vi "USB RAW - Bulk.vi"(6 "error in (no error)":errorcluster, 7 "Bulk Out Buffer":string="*IDN?\n", 8 "Bytes To Read":u32=512, 9 "USB RAW VISA resource name":refnum<visa-resource-name>) -> (0 "error out":errorcluster, 2 "Bulk In Buffer":string)   [LabVIEW 2012]
doc: "This example shows how to read and write simple user events from and to a USB RAW device. \n\n<b>Note:</b> This example works only with USB RAW devices.\n\nBefore you run this VI, install a USB RAW device and configure NI Measurement & Automation Explorer (MAX) to recognize the USB device. You can read to and write from the USB RAW device only after you install and configure the USB RAW device and open a session to the device. To read to or write from another device, close the session to the current device, select another device from the <b>USB RAW VISA resource name</b> pull-down menu, and open a session to the new device. \n\nWhen you complete the read or write, click the <b>Stop</b> button to stop the VI."
panel:
  in  "Clear 2":bool
  in  "Stop":bool
  in  "Clear":bool
  in  "BulkIn":bool
  in  "BulkOut":bool
  in  "CloseSession":bool
  in  "OpenSession":bool
  # "On Windows/Linux, consider using the Instrument Driver Finder (Help>>Find Instrument Drivers) to search for an instrument driver for your instrument."
  # "Select Help>>Show Context Help and move the cursor over the VI icon to display help for this VI."
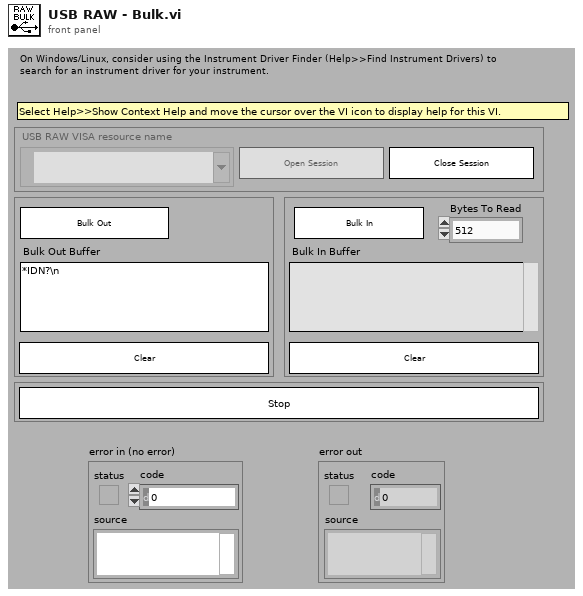
[diagram p1: front panel]
types:
  T1 = enum16{"Initialize/Session Closed", "Session Opened", "Do Nothing"}
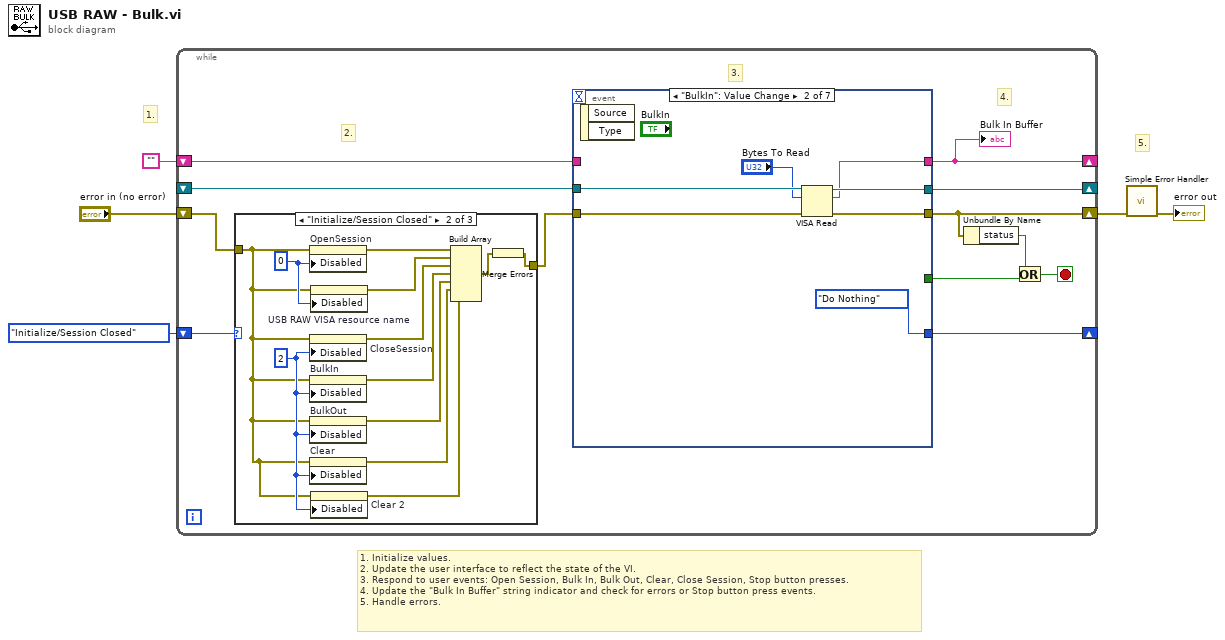
[diagram p0: block diagram]
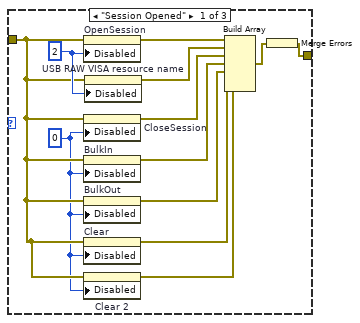
[diagram p2: hidden frame]
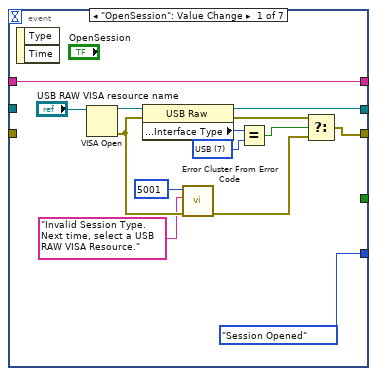
[diagram p4: hidden frame]
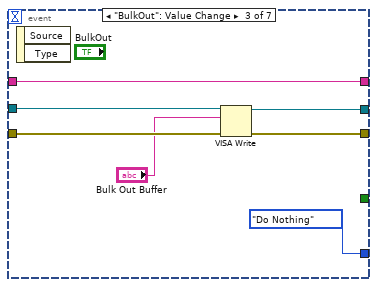
[diagram p5: hidden frame]
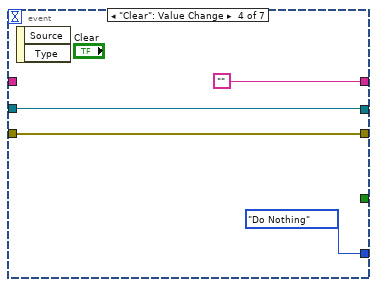
[diagram p6: hidden frame]
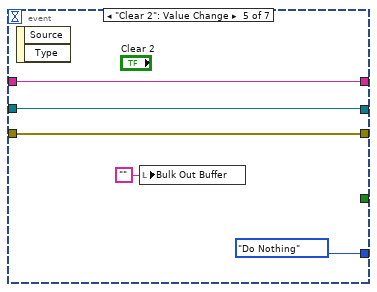
[diagram p7: hidden frame]
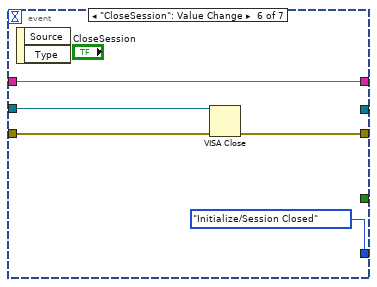
[diagram p8: hidden frame]
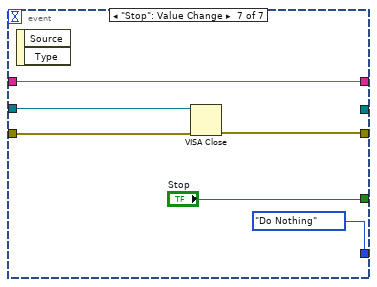
[diagram p9: hidden frame]
diagram:
  # "5."
  # "1."
  # "1. Initialize values.\n2. Update the user interface to reflect the state of the VI.\n3. Respond to user events: Open Session, Bulk In, Bulk Out, Clear, Close Session, Stop button presses.\n4. Update the \"Bulk In Buffer\" string indicator and check for errors or Stop button press events.\n5. Handle errors."
  n1 = while {
    shift-right: [w15] -> _
    shift-left: "" -> [w17]
    shift-right: [w16] -> w3
    shift-left: "error in (no error)" -> [w7]
    shift-right: [w11] -> _
    shift-left: _ -> [w10]
    shift-right: [w6] -> _
    shift-left: T1."Initialize/Session Closed" -> [w9]
    stop <- w12 stop-if-true
    # "4."
    # "3."
    # "2."
    n2 = case shown="\"Initialize/Session Closed\"" w9 {
      tunnel: [w27 w39 w42] -> w8
      tunnel: w7 -> [w20 w31 w42]
      frame "Session Opened" {
        w18 = u8 0 ("Disabled")
        w26 = u8 2 ("Disabled")
        n3 = property on="OpenSession" class="Bool"(error in=w20, "Disabled"=w26) -> (error out=w28:errorcluster)  [unwired: 1 in, 1 out]
        n4 = property on="CloseSession" class="Bool"(error in=w20, "Disabled"=w18) -> (error out=w24:errorcluster)  [unwired: 1 in, 1 out]
        n5 = property on="BulkIn" class="Bool"(error in=w20, "Disabled"=w18) -> (error out=w23:errorcluster)  [unwired: 1 in, 1 out]
        n6 = property on="BulkOut" class="Bool"(error in=w20, "Disabled"=w18) -> (error out=w22:errorcluster)  [unwired: 1 in, 1 out]
        n7 = property on="Clear" class="Bool"(error in=w20, "Disabled"=w18) -> (error out=w21:errorcluster)  [unwired: 1 in, 1 out]
        n8 = property on="Clear 2" class="Bool"(error in=w20, "Disabled"=w18) -> (error out=w19:errorcluster)  [unwired: 1 in, 1 out]
        n9 = property on="USB RAW VISA resource name" class="VISAName"(error in=w20, "Disabled"=w26) -> (error out=w25:errorcluster)  [unwired: 1 in, 1 out]
        n10 = Build Array(w28, w25, w24, w23, w22, w21, w19) -> (w29:errorcluster[])
        n11 = Merge Errors(w29) -> (w27:errorcluster)
      }
      frame "Initialize/Session Closed" {
        w32 = u8 2 ("Disabled")
        w38 = u8 0 ("Disabled")
        n12 = property on="OpenSession" class="Bool"(error in=w31, "Disabled"=w38) -> (error out=w40:errorcluster)  [unwired: 1 in, 1 out]
        n13 = property on="CloseSession" class="Bool"(error in=w31, "Disabled"=w32) -> (error out=w36:errorcluster)  [unwired: 1 in, 1 out]
        n14 = property on="BulkIn" class="Bool"(error in=w31, "Disabled"=w32) -> (error out=w35:errorcluster)  [unwired: 1 in, 1 out]
        n15 = property on="BulkOut" class="Bool"(error in=w31, "Disabled"=w32) -> (error out=w34:errorcluster)  [unwired: 1 in, 1 out]
        n16 = property on="Clear" class="Bool"(error in=w31, "Disabled"=w32) -> (error out=w33:errorcluster)  [unwired: 1 in, 1 out]
        n17 = property on="USB RAW VISA resource name" class="VISAName"(error in=w31, "Disabled"=w38) -> (error out=w37:errorcluster)  [unwired: 1 in, 1 out]
        n18 = property on="Clear 2" class="Bool"(error in=w31, "Disabled"=w32) -> (error out=w30:errorcluster)  [unwired: 1 in, 1 out]
        n19 = Build Array(w40, w37, w36, w35, w34, w33, w30) -> (w41:errorcluster[])
        n20 = Merge Errors(w41) -> (w39:errorcluster)
      }
      frame "Do Nothing", Default {
      }
    }
    n21 = event shown="[1] \"BulkIn\": Value Change" {
      selector: _ -> [_ _ _ _ _ _ _]
      dyn-events: _ -> [_ _ _ _ _ _ _]
      timeout: _ -> [_ _ _ _ _ _ _]
      tunnel: [_ _ _ _ _ _ "Stop"] -> w13
      tunnel: [w56 w61 w70 "" w75 w84 w89] -> w15
      tunnel: w17 -> [w56 _ w70 _ w75 w84 w89]
      tunnel: [w50 w63 w67 w73 w79 w80 w85] -> w16
      tunnel: w8 -> [_ w59 w68 w73 w79 w81 w86]
      tunnel: [w52 w62 w66 w72 w78 _ _] -> w11
      tunnel: w10 -> [_ w60 w69 w72 w78 w82 w87]
      tunnel: [T1."Session Opened" T1."Do Nothing" T1."Do Nothing" T1."Do Nothing" T1."Do Nothing" T1."Initialize/Session Closed" T1."Do Nothing"] -> w6
      event "OpenSession": Value Change {
        w48 = u16 7 items=["GPIB"=1, "VXI"=2, "GPIB-VXI"=3, "Serial"=4, "PXI"=5, "TCPIP"=6, "USB"=7] ("Interface Information:Interface Type")
        n22 = event-data() -> ()  [unwired: 3 out]
        n23 = VISA Open(VISA resource name="USB RAW VISA resource name") -> (VISA resource name=w53:refnum<visa-resource-name>, error out=w46:errorcluster)  [unwired: 1 in, 3 out]
        n24 = property class="USB Raw"(reference=w53, error in=w46) -> (reference out=w52:refnum<visa-resource-name>, error out=w51:errorcluster, "Interface Information:Interface Type"=w49:u16)
        n25 = call <vilib>:"Error Cluster From Error Code.vi"("error in (no error)"=w46, "error message (\"\")"="Invalid Session Type.  Next time, select a USB RAW VISA Resource." ("error message (\"\")"), "error code (0)"=5001) -> ("error out"=w43:errorcluster)  [unwired: 1 in, 5 out]
        n26 = Equal?(x=w49, y=w48) -> (x = y?=w47:bool)
        n27 = Select(t=w51, s=w47, f=w43) -> (s? t:f=w50:errorcluster)
      }
      event "BulkIn": Value Change {
        n28 = event-data() -> ()  [unwired: 3 out]
        n29 = VISA Read(VISA resource name=w60, byte count="Bytes To Read", error in (no error)=w59) -> (VISA resource name out=w62:refnum<visa-resource-name>, read buffer=w61:string, error out=w63:errorcluster)  [unwired: 1 out]
      }
      event "BulkOut": Value Change {
        n30 = event-data() -> ()  [unwired: 3 out]
        n31 = VISA Write(VISA resource name=w69, write buffer="Bulk Out Buffer", error in (no error)=w68) -> (VISA resource name out=w66:refnum<visa-resource-name>, error out=w67:errorcluster)  [unwired: 1 out]
      }
      event "Clear": Value Change {
        n32 = event-data() -> ()  [unwired: 3 out]
      }
      event "Clear 2": Value Change {
        n33 = event-data() -> ()  [unwired: 3 out]
        n34 = local write "Bulk Out Buffer"("") -> ()
      }
      event "CloseSession": Value Change {
        n35 = event-data() -> ()  [unwired: 3 out]
        n36 = VISA Close(VISA resource name=w82, error in (no error)=w81) -> (error out=w80:errorcluster)
      }
      event "Stop": Value Change {
        n37 = event-data() -> ()  [unwired: 3 out]
        n38 = VISA Close(VISA resource name=w87, error in (no error)=w86) -> (error out=w85:errorcluster)
      }
    }
    "Bulk In Buffer" <- w15
    n39 = Unbundle By Name(w16) -> ("status"=w14:bool)
    n40 = Or(x=w14, y=w13) -> (x .or. y?=w12:bool)
  }
  n41 = call <vilib>:"Simple Error Handler.vi"("error in (no error)"=w3) -> ("error out"=→"error out":errorcluster)  [unwired: 1 in, 7 out]
